vi "ItoB.vi"(11 "Current":dbl) -> (3 "Field":dbl)   [LabVIEW 2013]
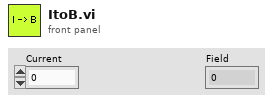
[diagram p1: front panel]
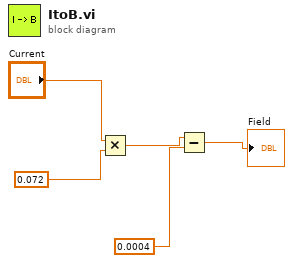
[diagram p0: block diagram]
diagram:
  n1 = Multiply(x="Current", y=0.072) -> (x*y=w3:dbl)
  n2 = Subtract(x=w3, y=0.0004) -> (x-y=→"Field":dbl)
